vi "Export Single VI Help.vi"(6 "Show FP":bool, 8 "error in (no error)":errorcluster, 10 "VI Description":string, 11 "Path":path) -> (0 "error out":errorcluster, 2 "VI Description Out":string)   [LabVIEW 2017, in "csmdoc.lvlib"]
uses:
  csmdoc.lvlib
  _tool/_file/csm-file-support.lvlib
  Communicable State Machine.lvlib
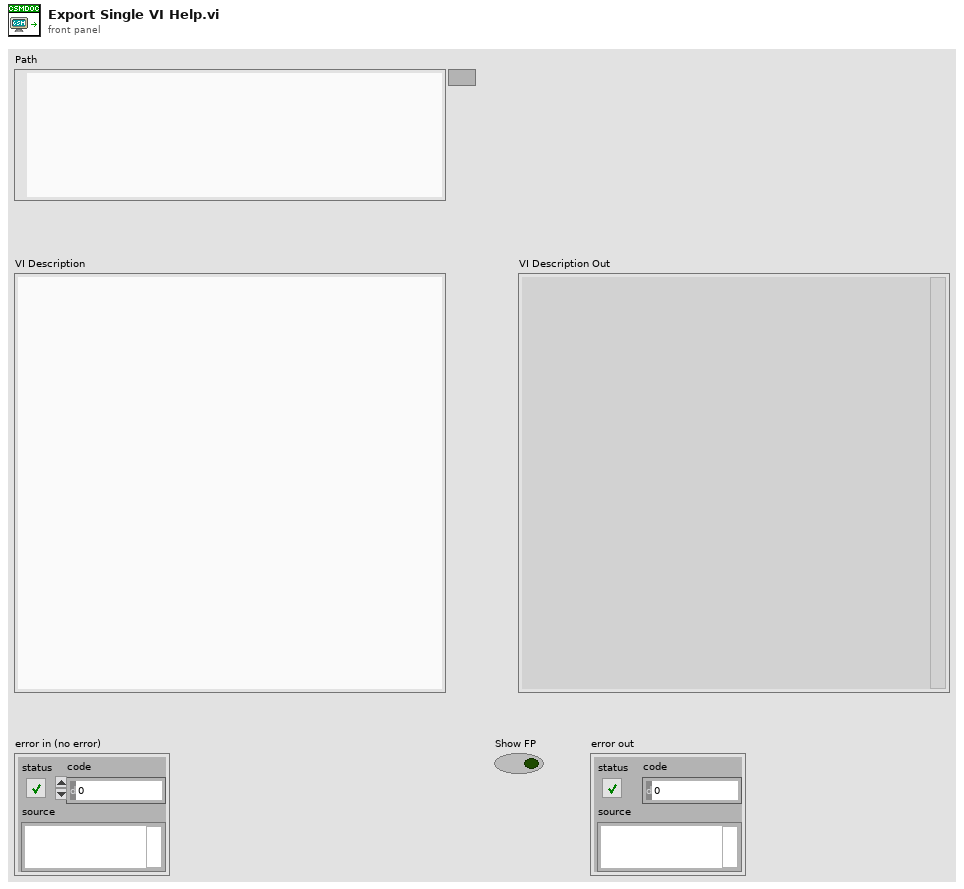
[diagram p1: front panel]
types:
  T1 = typedef "csmdoc.lvlib/DocNote.ctl" = cluster{"ID":string, "Content":string, "Type":string}
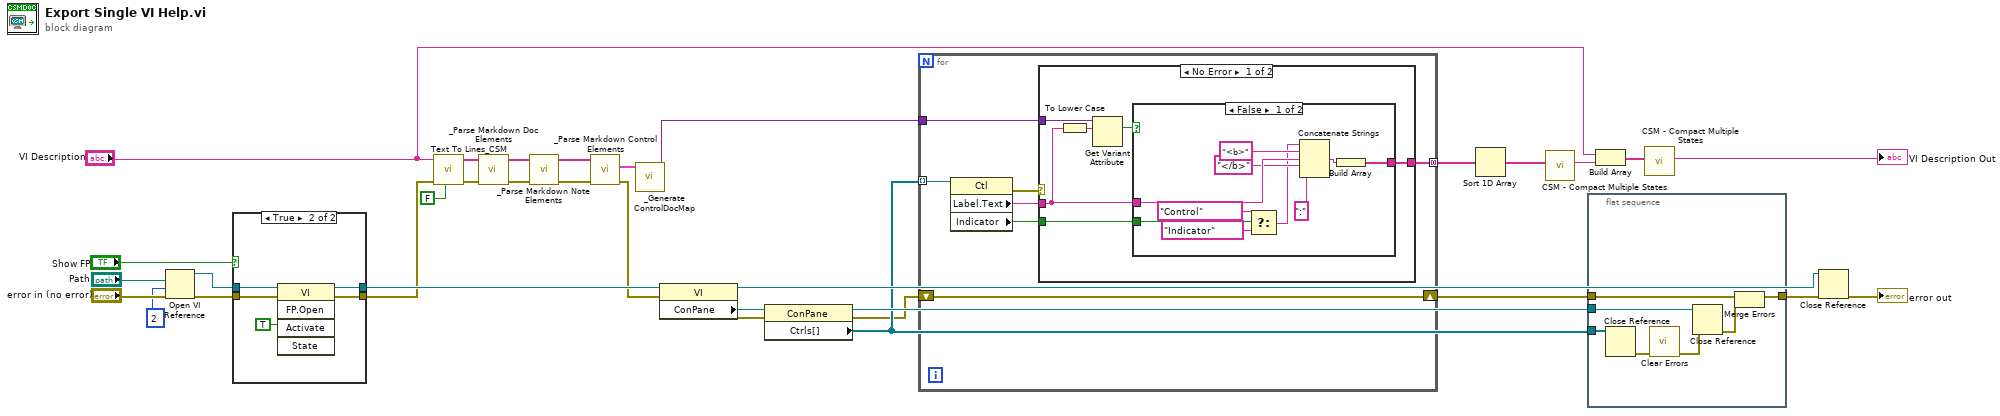
[diagram p0: block diagram]
diagram:
  n1 = Open VI Reference(vi path="Path", options=2, error in (no error)="error in (no error)") -> (vi reference=w27:refnum<vi>, error out=w28:errorcluster)  [unwired: 3 in]
  n2 = case shown="True" "Show FP" {
    tunnel: w28 -> [w34 w39]
    tunnel: w27 -> [w35 w38]
    tunnel: [w34 w37] -> w20
    tunnel: [w35 w36] -> w21
    frame False {
    }
    frame True {
      n3 = invoke class="VI" method="FP.Open"(reference=w38, error in=w39, "Activate"=TRUE ("Activate?")) -> (reference out=w36:refnum<vi>, error out=w37:errorcluster)  [unwired: 2 in, 3 out]
    }
  }
  n4 = call "Text To Lines_CSM.vi"("Remove Empty Lines? (T)"=FALSE ("Remove Empty Lines?(T)"), "error in (no error)"=w20, "String"="VI Description") -> ("error out"=w24:errorcluster, "Lines"=w25:string[])  [unwired: 7 in]
  n5 = call "_Parse Markdown Doc Elements.vi"("Error in"=w24, "Lines"=w25) -> ("Error out"=w22:errorcluster, "Lines (dup)"=w23:string[])  [unwired: 7 in, 1 out]
  n6 = call "_Parse Markdown Note Elements.vi"("Error in"=w22, "Lines"=w23) -> ("Error out"=w3:errorcluster, "Lines (dup)"=w4:string[])  [unwired: 7 in, 1 out]
  n7 = call "_Parse Markdown Control Elements.vi"("Error in"=w3, "Lines"=w4) -> ("Error out"=w2:errorcluster, "Array"=w5:T1[])  [unwired: 7 in, 1 out]
  n8 = call "_Generate ControlDocMap.vi"("Array"=w5) -> ("Variant"=w1:variant)  [unwired: 10 in]
  n9 = property class="VI"(reference=w21, error in=w2) -> (reference out=w16:refnum<vi>, error out=w18:errorcluster, "ConPane"=w19:refnum<vi>)
  n10 = property class="ConPane"(reference=w19, error in=w18) -> (reference out=w17:refnum<vi>, error out=w7:errorcluster, "Ctrls[]"=w14:refnum<vi>[])
  n11 = for {
    tunnel: w1 -> [w46]
    tunnel: w14 -> [w47] mode=indexing
    tunnel: [w43] -> w13 mode=concatenating
    shift-right: [w42] -> w8
    shift-left: w7 -> [w42]
    n12 = property class="Ctl"(reference=w47) -> (error out=w41:errorcluster, "Label.Text"=w45:string, "Indicator"=w44:bool)  [unwired: 1 in, 1 out]
    n13 = case shown="No Error" w41 {
      tunnel: w46 -> [w53 _]
      tunnel: w45 -> [w51 _]
      tunnel: w44 -> [w50 _]
      tunnel: [w49 _] -> w43
      frame No Error {
        n14 = To Lower Case(string=w51) -> (all lower case string=w48:string)
        n15 = Get Variant Attribute(Variant=w53, name=w48) -> (found=w52:bool)  [unwired: 2 in, 3 out]
        n16 = case shown="False" w52 {
          tunnel: w51 -> [w63 _]
          tunnel: w50 -> [w58 _]
          tunnel: [w59 _] -> w49
          frame False {
            n17 = Select(t="Control" ("string"), s=w58, f="Indicator" ("string")) -> (s? t:f=w54:string)
            n18 = Concatenate Strings(w54, "<b>" ("string"), w63, "</b>" ("string"), ":" ("string")) -> (w60:string)
            n19 = Build Array(w60) -> (w59:string[])
          }
          frame True {
          }
        }
      }
      frame Error {
      }
    }
  }
  n20 = Sort 1D Array(array=w13) -> (sorted array=w6:string[])
  n21 = call "CSM - Compact Multiple States.vi"("Multiple States"=w6) -> ("States"=w12:string)  [unwired: 9 in]
  n22 = flat-sequence {
    tunnel: w14 -> [w70]
    tunnel: w17 -> [w69]
    tunnel: [w67] -> w15
    tunnel: w8 -> [w65]
    frame #0 {
      n23 = Close Reference(reference=w70) -> (error out=w68:errorcluster)  [unwired: 1 in]
      n24 = call <vilib>:"Clear Errors.vi"("error in (no error)"=w68) -> ("error out"=w64:errorcluster)  [unwired: 5 in, 1 out]
      n25 = Close Reference(reference=w69, error in (no error)=w64) -> (error out=w66:errorcluster)
      n26 = Merge Errors(w65, w66) -> (w67:errorcluster)
    }
  }
  n27 = Build Array("VI Description", w12) -> (w10:string[])
  n28 = call "CSM - Compact Multiple States.vi"("Multiple States"=w10) -> ("States"=→"VI Description Out":string)  [unwired: 9 in]
  n29 = Close Reference(reference=w16, error in (no error)=w15) -> (error out=→"error out":errorcluster)
